vi "Configure Zone.vi"(0 "VISA resource name":refnum<visa-resource-name>, 1 "Output (0)":i32 min=0 max=1 step=1, 2 "Zone (1)":i32=1 min=1 max=10 step=1, 3 "Upper Bound (0.00000E+0)":dbl min=0.0 max=100000000.0 step=1e-06 format="%^.5e", 4 "Heater Manual Output (%)":dbl min=-100.0 max=100.0 step=0.001 format="%.3f", 5 "error in (no error)":errorcluster, 6 "P Value (10.000)":dbl=10.0 min=0.0 max=1000.0 step=0.001 format="%.3f", 7 "Heater Range (0: Off)":u16(ring) items=["Off", "31.6 uA", "100 uA", "316 uA", "1.00 mA", "3.16 mA", "10.0 mA", "31.6 mA", "100 mA"], 8 "I Value (20)":dbl=20.0 min=0.0 max=10000.0 step=1e-06, 9 "Ramp Rate (0)":dbl min=0.0 max=9999.0 step=1e-06 format="%.2f", 10 "D Value (0)":dbl min=0.0 max=2500.0 step=1e-06, 11 "Relay Low (0: Off)":u16(ring) items=["Off", "On"], 13 "Relay High (0: Off)":u16(ring) items=["Off", "On"]) -> (14 "VISA resource name out":refnum<visa-resource-name>, 19 "error out":errorcluster)   [LabVIEW 2019, in "Lake Shore 372.lvlib"]
doc: "Configures the parameters of the zone table. \n\nNotes:\nConfigures the control loop limit band parameters used in conjunction with the status byte register. Refer to section 6.2.6 in Model 372 Manual for further details."
uses:
  Lake Shore 372.lvlib
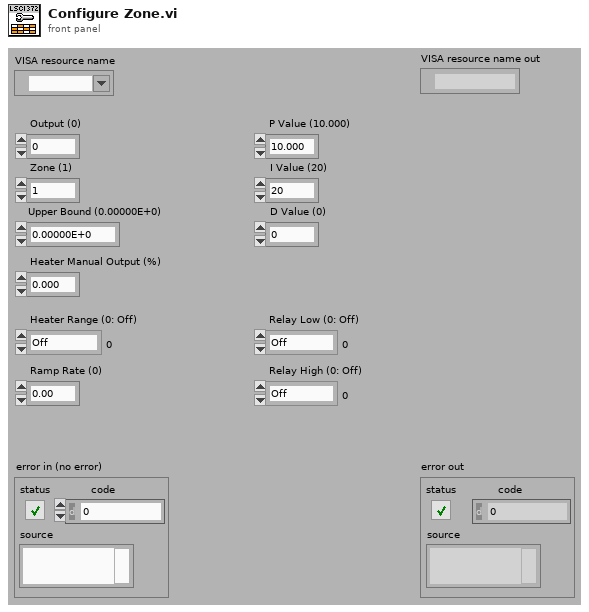
[diagram p1: front panel]
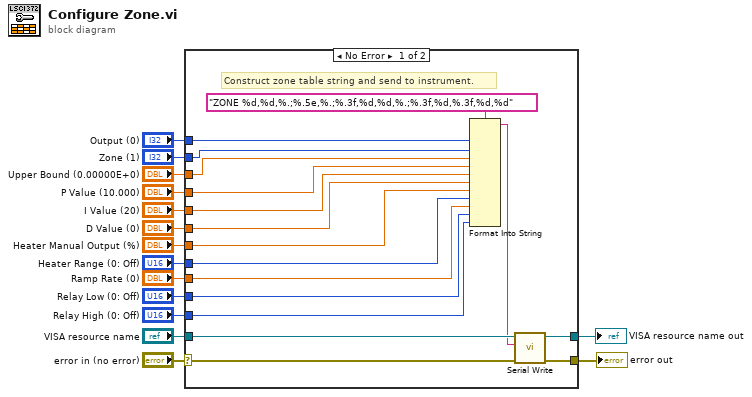
[diagram p0: block diagram]
diagram:
  n1 = case shown="No Error" "error in (no error)" {
    selector: "error in (no error)" -> [w28 w33]
    tunnel: [w32 w34] -> w15
    tunnel: [w31 w33] -> w14
    tunnel: "VISA resource name" -> [w30 w34]
    tunnel: "Output (0)" -> [w27 _]
    tunnel: "Zone (1)" -> [w26 _]
    tunnel: "Upper Bound (0.00000E+0)" -> [w25 _]
    tunnel: "P Value (10.000)" -> [w24 _]
    tunnel: "I Value (20)" -> [w23 _]
    tunnel: "D Value (0)" -> [w22 _]
    tunnel: "Heater Manual Output (%)" -> [w21 _]
    tunnel: "Heater Range (0: Off)" -> [w20 _]
    tunnel: "Ramp Rate (0)" -> [w19 _]
    tunnel: "Relay Low (0: Off)" -> [w18 _]
    tunnel: "Relay High (0: Off)" -> [w17 _]
    frame No Error {
      # "Construct zone table string and send to instrument."
      n2 = Format Into String(format string="ZONE %d,%d,%.;%.5e,%.;%.3f,%d,%d,%.;%.3f,%d,%.3f,%d,%d", w27, w26, w25, w24, w23, w22, w21, w20, w19, w18, w17) -> (resulting string=w16:string)  [unwired: 2 in, 1 out]
      n3 = call "Serial Write.vi"("error in (no error)"=w28, "Write Buffer (\"\")"=w16, "VISA resource name"=w30) -> ("error out"=w31:errorcluster, "VISA resource name out"=w32:refnum<visa-resource-name>)  [unwired: 6 in, 1 out]
    }
    frame Error {
    }
  }
  "VISA resource name out" <- w15
  "error out" <- w14
